vi "Browse_Disk_Sever.vi"(1 "Folder Hierarchy":string[](array[string])) -> (0 "Folders and files":T1(array[cluster]))   [LabVIEW 2012]
uses:
  Anemometry/Anemometry Sub Vis/Globals/Constants_global.vi
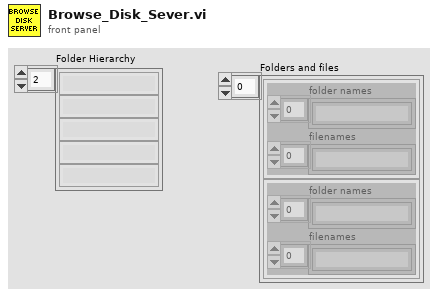
[diagram p1: front panel]
types:
  T1 = cluster{"folder names":string[], "filenames":string[]}[]
  T2 = cluster{"folder names":string[], "filenames":string[]}
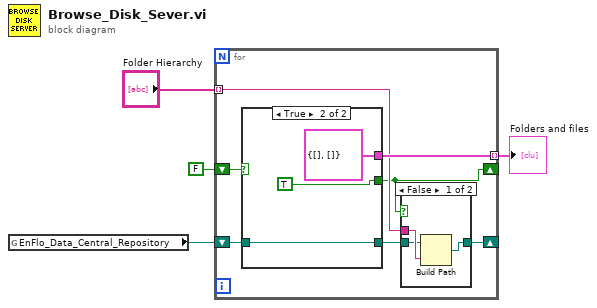
[diagram p0: block diagram]
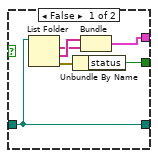
[diagram p3: hidden frame]
diagram:
  n1 = global read "Constants_global.vi" "EnFlo_Data_Central_Repository"() -> (w1:path)
  n2 = for {
    shift-right: [w6] -> _
    shift-left: w1 -> [w9]
    tunnel: [w11] -> w4 mode=indexing
    shift-right: [w5] -> _
    shift-left: FALSE -> [w10]
    tunnel: "Folder Hierarchy" -> [w8] mode=indexing
    n3 = case shown="True" w10 {
      tunnel: w9 -> [w16 w22]
      tunnel: [w16 w22] -> w7
      tunnel: [w19 T2 {"folder names"=[], "filenames"=[]}] -> w11
      tunnel: [w17 TRUE ("status")] -> w5
      frame False {
        n4 = List Folder(path=w16) -> (filenames=w20:string[], folder names=w21:string[], error out=w18:errorcluster)  [unwired: 3 in, 1 out]
        n5 = Unbundle By Name(w18) -> ("status"=w17:bool)
        n6 = Bundle("folder names"=w21, "filenames"=w20) -> (w19:T2)  [unwired: 1 in]
      }
      frame True {
      }
    }
    n7 = case shown="False" w5 {
      tunnel: w8 -> [w14 _]
      tunnel: w7 -> [w13 w15]
      tunnel: [w12 w15] -> w6
      frame False {
        n8 = Build Path(base path=w13, name or relative path=w14) -> (appended path=w12:path)
      }
      frame True {
      }
    }
  }
  "Folders and files" <- w4
